vi "Compact.vi"(11 "Flattened Data":string) -> (3 "Compacted":string)   [LabVIEW 2020, in "JSONtext.lvlib"]
doc: "Converts binary data into an encoded form that produces more compact JSON, by avoiding values that become \\uXXXX excapped codes."
uses:
  <vilib>/JDP Science/JSONtext/JSONtext.lvlib
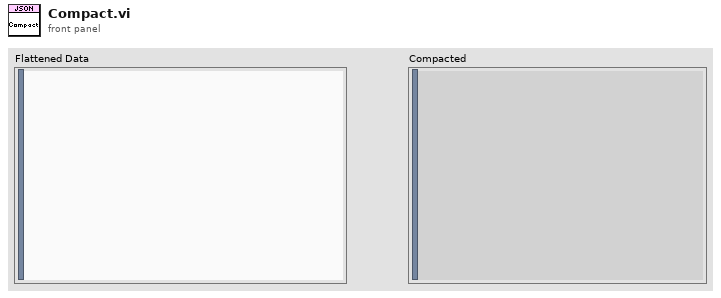
[diagram p1: front panel]
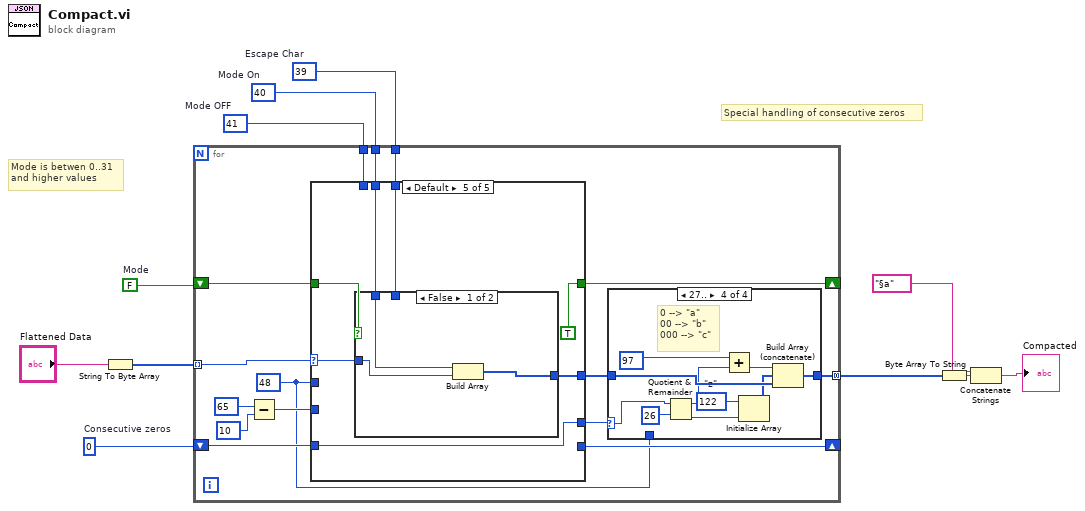
[diagram p0: block diagram]
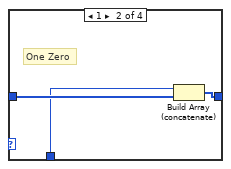
[diagram p3: hidden frame]
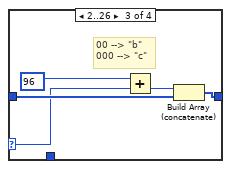
[diagram p4: hidden frame]
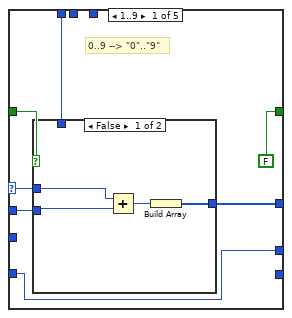
[diagram p5: hidden frame]
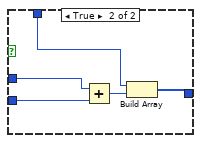
[diagram p6: hidden frame]
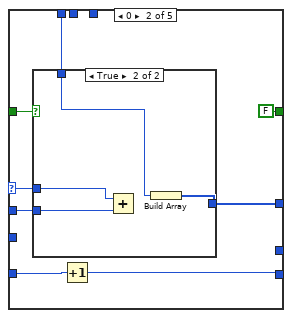
[diagram p7: hidden frame]
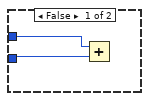
[diagram p8: hidden frame]
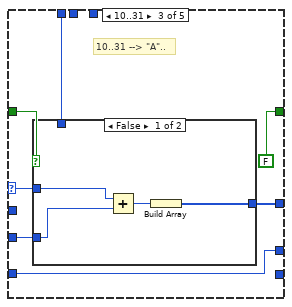
[diagram p9: hidden frame]
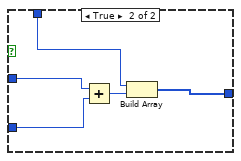
[diagram p10: hidden frame]
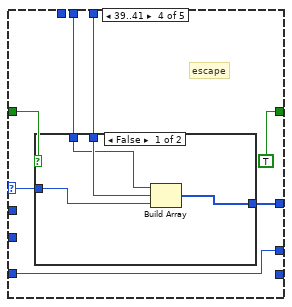
[diagram p11: hidden frame]
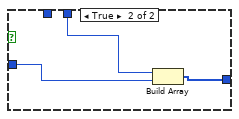
[diagram p12: hidden frame]
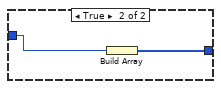
[diagram p13: hidden frame]
diagram:
  w1 = u32 0  # Consecutive zeros
  w10 = u8 41  # Mode OFF
  w9 = u8 40  # Mode On
  w8 = u8 39  # Escape Char
  w3 = FALSE  # Mode
  # "Special handling of consecutive zeros"
  # "Mode is betwen 0..31\nand higher values"
  n1 = String To Byte Array(string="Flattened Data") -> (unsigned byte array=w2:u8[])
  n2 = for {
    tunnel: w2 -> [w25] mode=indexing
    shift-right: [w23] -> _
    shift-left: w3 -> [w26]
    tunnel: [w14] -> w4 mode=concatenating
    tunnel: w8 -> [w22]
    tunnel: w9 -> [w21]
    tunnel: w10 -> [w20]
    shift-right: [w15] -> _
    shift-left: w1 -> [w16]
    w12 = u8 48 ("y")
    n3 = Subtract(x=u8 65 ("y"), y=u8 10) -> (x-y=w17:u8)
    n4 = case shown="Default" w25 {
      selector: w25 -> [w51 w68 w81 w97 w111]
      tunnel: w26 -> [w52 w69 w82 w98 w112]
      tunnel: [w50 w67 w80 w96 w110] -> w24
      tunnel: [FALSE FALSE FALSE TRUE TRUE] -> w23
      tunnel: w22 -> [_ _ _ w94 w108]
      tunnel: w21 -> [_ _ _ w93 w107]
      tunnel: w20 -> [w48 w65 w78 _ _]
      tunnel: w17 -> [_ _ w77 _ _]
      tunnel: w12 -> [w47 w64 _ _ _]
      tunnel: w16 -> [w46 w63 w76 w92 w106]
      tunnel: [_ w62 _ _ _] -> w15
      tunnel: [w46 _ w76 w92 w106] -> w13
      frame 1..9 {
        # "0..9 --> \"0\"..\"9\""
        n5 = case shown="False" w52 {
          tunnel: w51 -> [w56 w61]
          tunnel: [w54 w59] -> w50
          tunnel: w48 -> [_ w58]
          tunnel: w47 -> [w53 w57]
          frame False {
            n6 = Add(x=w56, y=w53) -> (x+y=w55:u8)
            n7 = Build Array(w55) -> (w54:u8[])
          }
          frame True {
            n8 = Add(x=w61, y=w57) -> (x+y=w60:u8)
            n9 = Build Array(w58, w60) -> (w59:u8[])
          }
        }
      }
      frame 0 {
        n10 = case shown="True" w69 {
          tunnel: w68 -> [w71 w75]
          tunnel: [_ w74] -> w67
          tunnel: w65 -> [_ w73]
          tunnel: w64 -> [w70 w72]
          frame False {
            n11 = Add(x=w71, y=w70) -> ()  [unwired: 1 out]
          }
          frame True {
            n12 = Add(x=w75, y=w72) -> ()  [unwired: 1 out]
            n13 = Build Array(w73) -> (w74:u8[])
          }
        }
        n14 = Increment(x=w63) -> (x+1=w62:u32)
      }
      frame 10..31 {
        # "10..31 --> \"A\".."
        n15 = case shown="False" w82 {
          tunnel: w81 -> [w86 w91]
          tunnel: [w84 w89] -> w80
          tunnel: w78 -> [_ w88]
          tunnel: w77 -> [w83 w87]
          frame False {
            n16 = Add(x=w86, y=w83) -> (x+y=w85:u8)
            n17 = Build Array(w85) -> (w84:u8[])
          }
          frame True {
            n18 = Add(x=w91, y=w87) -> (x+y=w90:u8)
            n19 = Build Array(w88, w90) -> (w89:u8[])
          }
        }
      }
      frame 39..41 {
        # "escape"
        n20 = case shown="False" w98 {
          tunnel: w97 -> [w101 w105]
          tunnel: [w102 w104] -> w96
          tunnel: w94 -> [w100 w103]
          tunnel: w93 -> [w99 _]
          frame False {
            n21 = Build Array(w99, w100, w101) -> (w102:u8[])
          }
          frame True {
            n22 = Build Array(w103, w105) -> (w104:u8[])
          }
        }
      }
      frame Default {
        n23 = case shown="False" w112 {
          tunnel: w111 -> [w115 w117]
          tunnel: [w114 w116] -> w110
          tunnel: w108 -> [_ _]
          tunnel: w107 -> [w113 _]
          frame False {
            n24 = Build Array(w113, w115) -> (w114:u8[])
          }
          frame True {
            n25 = Build Array(w117) -> (w116:u8[])
          }
        }
      }
    }
    n26 = case shown="27.." w13 {
      selector: w13 -> [_ _ w31 w36]
      tunnel: w24 -> [w27 w30 w35 w45]
      tunnel: [w27 w29 w34 w44] -> w14
      tunnel: w12 -> [_ w28 _ _]
      frame 0 {
      }
      frame 1 {
        # "One Zero"
        n27 = Build Array (concatenate)(w28, w30) -> (w29:u8[])
      }
      frame 2..26 {
        # "00 --> \"b\"\n000 --> \"c\""
        n28 = Add(x=u8 96 ("y"), y=w31) -> (x+y=w33:u32)
        n29 = Build Array (concatenate)(w33, w35) -> (w34:u32[])
      }
      frame 27.. {
        w38 = u8 122  # "z"
        # "0 --> \"a\"\n00 --> \"b\"\n000 --> \"c\""
        n30 = Quotient & Remainder(x=w36, y=u8 26) -> (x-y*floor(x/y)=w40:u32, floor(x/y)=w39:u32)
        n31 = Add(x=u8 97 ("y"), y=w40) -> (x+y=w43:u32)
        n32 = Initialize Array(w38, w39) -> (w37:u8[])
        n33 = Build Array (concatenate)(w43, w37, w45) -> (w44:u32[])
      }
    }
  }
  n34 = Byte Array To String(unsigned byte array=w4) -> (string=w5:string)
  n35 = Concatenate Strings("§a" ("string"), w5) -> (→"Compacted":string)
